vi "Fetch Waveform Measurement (Histogram).vi"(0 "VISA resource name":refnum<visa-resource-name>, 7 "Function (0:Wfm Ct)":u16(ring) items=["Wfm Ct", "Median", "Pk-Pk", "Hits in Box", "Max", "Mean", "Peak Hits", "Min", "St Dev", "Sigma1", "Sigma2", "Sigma3"], 11 "error in (no error)":errorcluster) -> (4 "VISA resource name out":refnum<visa-resource-name>, 6 "Measurement":dbl, 15 "error out":errorcluster)   [LabVIEW 2011, in "Tektronix 7000 Series.lvlib"]
doc: "Initiates a waveform acquisition on the specified <B>Channel</B> and returns a <B>Measurement</B> value. Use the Fetch Waveform Measurement VI separately for any other waveform measurement on a channel without initiating another acquisition."
uses:
  Tektronix 7000 Series.lvlib
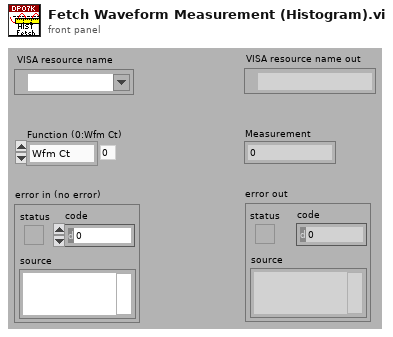
[diagram p1: front panel]
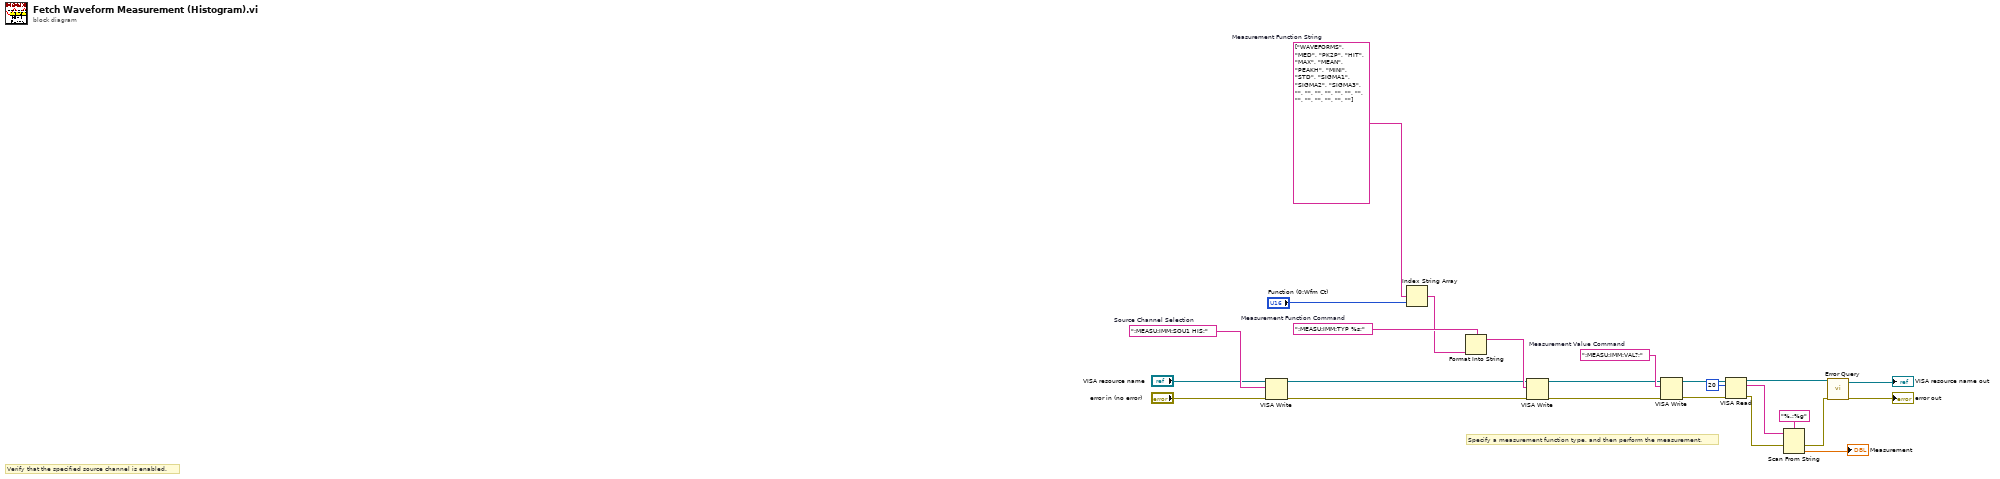
[diagram p0: block diagram]
diagram:
  w8 = ":MEASU:IMM:SOU1 HIS;"  # Source Channel Selection
  w20 = ":MEASU:IMM:VAL?;"  # Measurement Value Command
  w23 = ":MEASU:IMM:TYP %s;"  # Measurement Function Command
  w24 = string[] ["WAVEFORMS", "MED", "PK2P", "HIT", "MAX", "MEAN", "PEAKH", "MINI", "STD", "SIGMA1", "SIGMA2", "SIGMA3", "", "", "", "", "", "", "", "", "", "", "", "", ""]  # Measurement Function String
  # "Specify a measurement function type, and then perform the measurement."
  # "Verify that the specified source channel is enabled."
  n1 = VISA Write(VISA resource name="VISA resource name", write buffer=w8, error in (no error)="error in (no error)") -> (VISA resource name out=w11:refnum<visa-resource-name>, error out=w10:errorcluster)  [unwired: 1 out]
  n2 = Index String Array(1:"Function (0:Wfm Ct)", 2:w24) -> (0:w22:string)  [unwired: 1 in]
  n3 = Format Into String(format string=w23, w22) -> (resulting string=w21:string)  [unwired: 2 in, 1 out]
  n4 = VISA Write(VISA resource name=w11, write buffer=w21, error in (no error)=w10) -> (VISA resource name out=w13:refnum<visa-resource-name>, error out=w12:errorcluster)  [unwired: 1 out]
  n5 = VISA Write(VISA resource name=w13, write buffer=w20, error in (no error)=w12) -> (VISA resource name out=w19:refnum<visa-resource-name>, error out=w18:errorcluster)  [unwired: 1 out]
  n6 = VISA Read(VISA resource name=w19, byte count=u32 20, error in (no error)=w18) -> (VISA resource name out=w5:refnum<visa-resource-name>, read buffer=w16:string, error out=w2:errorcluster)  [unwired: 1 out]
  n7 = Scan From String(format string="%.;%g", input string=w16, error in=w2) -> (error out=w1:errorcluster, output 1=→"Measurement":dbl)  [unwired: 2 in, 2 out]
  n8 = call "Error Query.vi"("error in (no error)"=w1, "VISA resource name"=w5) -> ("error out"=→"error out":errorcluster, "VISA resource name out"=→"VISA resource name out":refnum<visa-resource-name>)  [unwired: 6 in, 2 out]
